vi "Set Magnet.vi"(4 "Mode":T2, 6 "Axis":T1=enum."Z", 8 "error in (no error)":errorcluster, 9 "Target Rate (T/min)":dbl, 10 "Target Field (T)":dbl, 11 "Instrument.Cryostat in":refnum<class "Instrument.Cryostat.lvclass">) -> (0 "error out":errorcluster, 3 "Instrument.Cryostat out":refnum<class "Instrument.Cryostat.lvclass">)   [LabVIEW 2019, in "Instrument.Cryostat.lvclass"]
uses:
  Instrument.Cryostat.lvclass
  Typedefs/Magnet Mode--Enum.ctl
  Typedefs/Magnet Axis--Enum.ctl
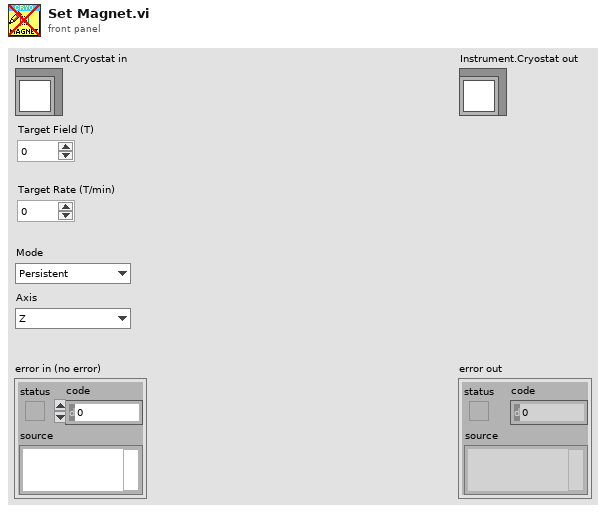
[diagram p1: front panel]
types:
  T1 = typedef "Instrument.Cryostat.lvclass/Magnet Axis--Enum.ctl" = enum16{"X", "Y", "Z"}
  T2 = typedef "Instrument.Cryostat.lvclass/Magnet Mode--Enum.ctl" = enum16{"Persistent", "Driven"}
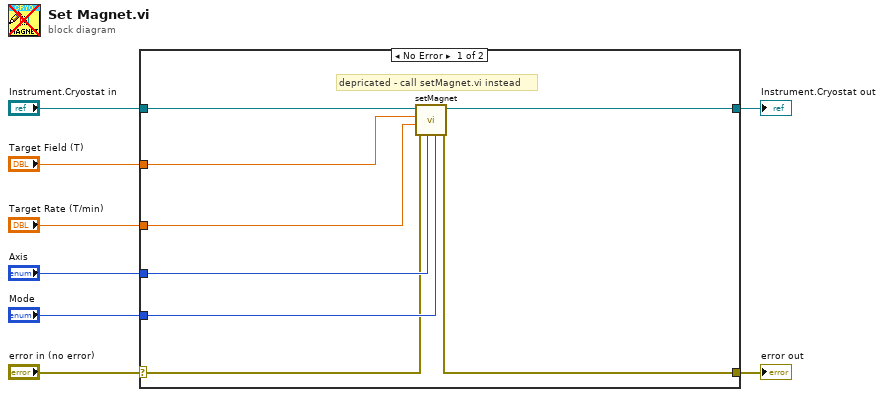
[diagram p0: block diagram]
diagram:
  n1 = case shown="No Error" "error in (no error)" {
    selector: "error in (no error)" -> [w12 w18]
    tunnel: [w11 w18] -> w7
    tunnel: [w16 w17] -> w5
    tunnel: "Instrument.Cryostat in" -> [w15 w17]
    tunnel: "Target Field (T)" -> [w9 _]
    tunnel: "Target Rate (T/min)" -> [w10 _]
    tunnel: "Axis" -> [w14 _]
    tunnel: "Mode" -> [w13 _]
    frame No Error {
      # "depricated - call setMagnet.vi instead"
      n2 = call-dynamic "setMagnet.vi"("Mode"=w13, "Axis"=w14, "error in (no error)"=w12, "Target Rate (T/min)"=w10, "Target Field (T)"=w9, "Instrument.Cryostat in"=w15) -> ("error out"=w11:errorcluster, "Instrument.Cryostat out"=w16:refnum<class "Instrument.Cryostat.lvclass">)  [unwired: 4 in]
    }
    frame Error {
    }
  }
  "error out" <- w7
  "Instrument.Cryostat out" <- w5
